vi "Copy All Data.vi"(8 "error in (no error)":errorcluster, 10 "src":refnum<class "Button.lvclass">, 11 "dest":refnum<class "Button.lvclass">) -> (0 "error out":errorcluster, 3 "object out":refnum<class "Button.lvclass">)   [LabVIEW 2012, in "Button.lvclass"]
doc: "Copy All the private data from src to destination"
uses:
  Button.lvclass
  Button.lvclass/Button.ctl
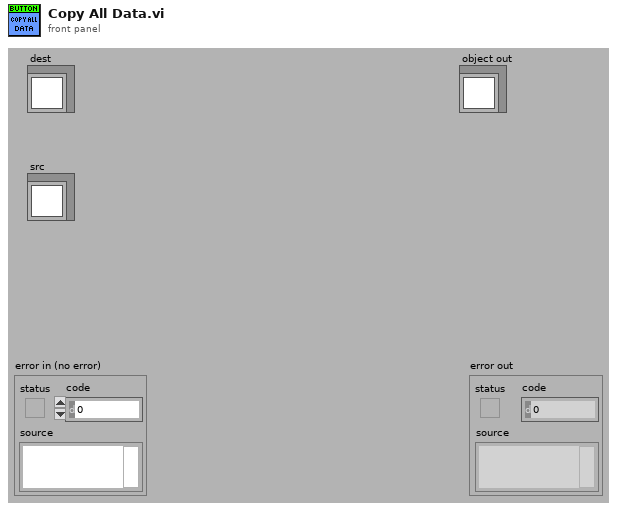
[diagram p1: front panel]
types:
  T1 = typedef "Button.lvclass/Button Type.ctl" = enum16{"Transitory", "Latching"}
  T2 = typedef "Button.lvclass/Button Status.ctl" = enum16{"Off", "Hover", "On", "Disabled"}
  T3 = typedef "imagedata.ctl" = cluster{"image type":i32, "image depth":i32, "image":u8[], "mask":u8[], "colors":u32[], "Rectangle":cluster{"left":i16, "top":i16, "right":i16, "bottom":i16}}
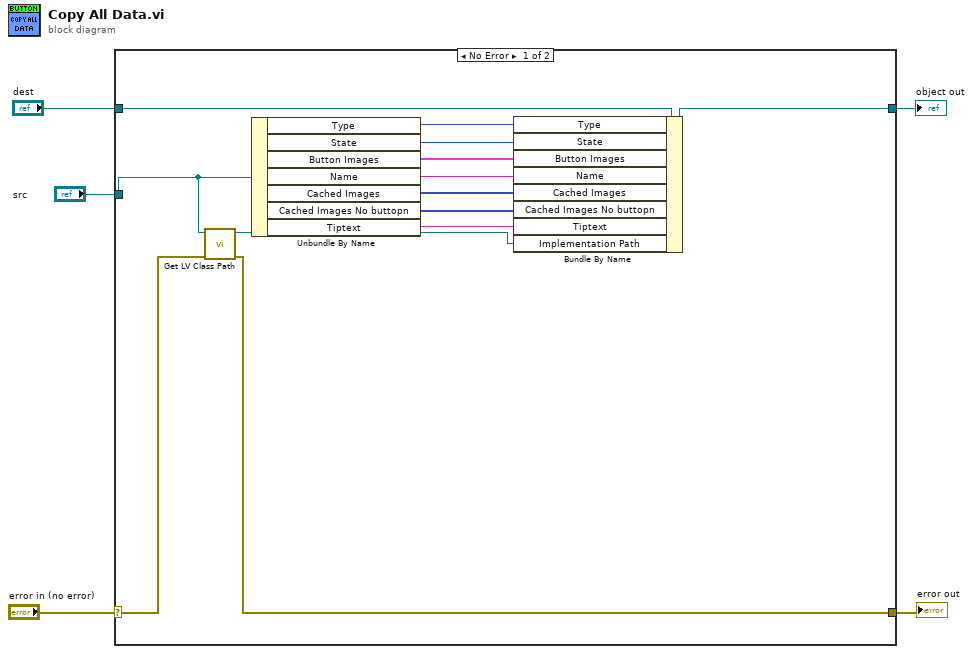
[diagram p0: block diagram]
diagram:
  n1 = case shown="No Error" "error in (no error)" {
    selector: "error in (no error)" -> [w7 w20]
    tunnel: [w6 w20] -> w4
    tunnel: [w17 w19] -> w2
    tunnel: "dest" -> [w18 w19]
    tunnel: "src" -> [w16 _]
    frame No Error {
      n2 = call <vilib>:"Get LV Class Path.vi"("error in (no error)"=w7, "object"=w16) -> ("error out"=w6:errorcluster, "class path"=w15:path)  [unwired: 8 in]
      n3 = Unbundle By Name(w16) -> ("Type"=w8:T1, "State"=w9:T2, "Button Images"=w10:T3[], "Name"=w11:string, "Cached Images"=w12:picture[], "Cached Images No buttopn"=w13:picture[], "Tiptext"=w14:string)
      n4 = Bundle By Name(cluster=w18, "Type"=w8, "State"=w9, "Button Images"=w10, "Name"=w11, "Cached Images"=w12, "Cached Images No buttopn"=w13, "Tiptext"=w14, "Implementation Path"=w15) -> (w17:refnum<class "Button.lvclass">)
    }
    frame Error {
    }
  }
  "error out" <- w4
  "object out" <- w2
